vi "GetQuackingLvclass.vi"(8 "error in (no error)":errorcluster, 11 "object in":refnum<class "Duck.lvclass">) -> (0 "error out":errorcluster, 2 "Quacking Behaviors.lvclass":refnum<class "Quacking Behaviors.lvclass">, 3 "object out":refnum<class "Duck.lvclass">)   [LabVIEW 2021, in "Duck.lvclass"]
uses:
  Duck.lvclass
  Quacking Behaviors/Quacking Behaviors.lvclass
  Duck.lvclass/Duck.ctl
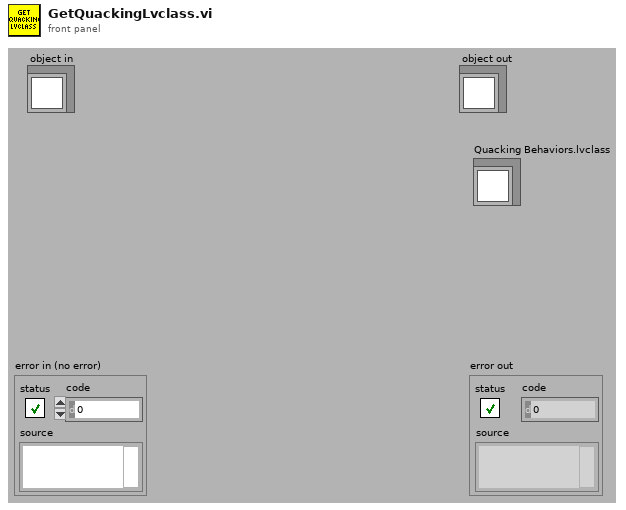
[diagram p1: front panel]
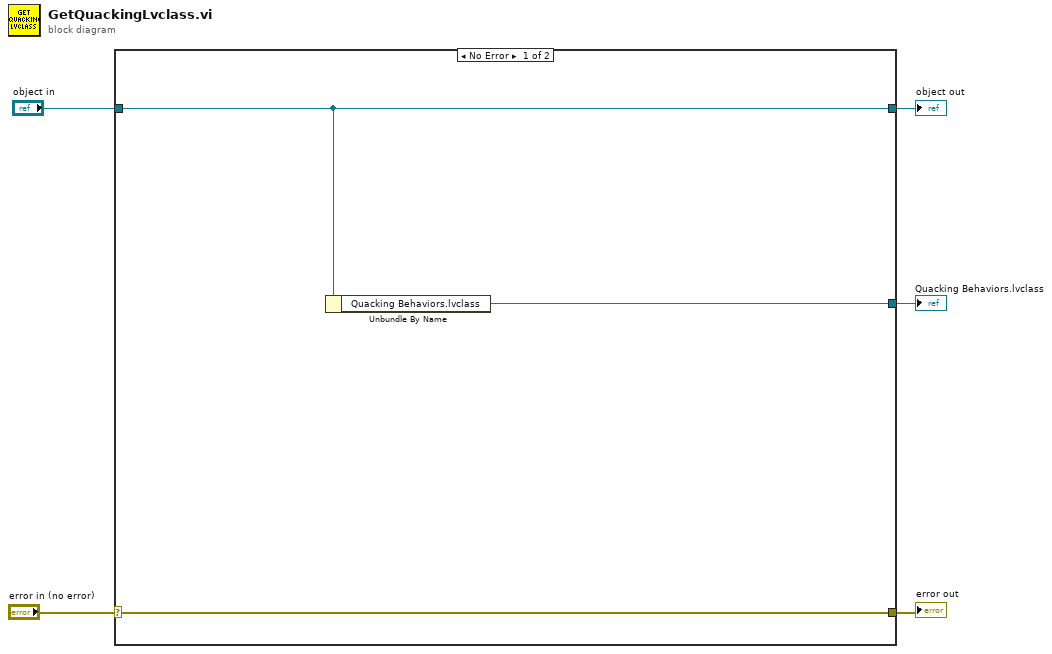
[diagram p0: block diagram]
diagram:
  n1 = case shown="No Error" "error in (no error)" {
    selector: "error in (no error)" -> [w7 w10]
    tunnel: [w7 w10] -> w4
    tunnel: [w6 w9] -> w2
    tunnel: "object in" -> [w6 w9]
    tunnel: [w8 _] -> w1
    frame No Error {
      n2 = Unbundle By Name(w6) -> ("Quacking Behaviors.lvclass"=w8:refnum<class "Quacking Behaviors.lvclass">)
    }
    frame Error {
    }
  }
  "error out" <- w4
  "object out" <- w2
  "Quacking Behaviors.lvclass" <- w1
